vi "Dashboard.vi"() -> ()   [LabVIEW 2021]
uses:
  <vilib>/Instr/_visa.llb/VISA Configure Serial Port (Instr).vi
  <vilib>/addons/database/Connection.llb/DB Tools Open Connec (Path).vi
  <vilib>/addons/database/NI_Database_API.lvlib
panel:
  in  "Controle do alarme":dbl
  out "Alta Temperatura":bool
  out "TEMPERATURA [ºC]":dbl
  out "Temperatura":dbl(graph)
  out "ACELERADOR":dbl(graph)
  out "FREIO":dbl(graph)
  out "Temperatura":dbl(knob) caption="Meter" scale=0.0..120.0
  out "FREIO":u8(slide) scale=0.0..100.0
  out "ACELERADOR":u8(slide) scale=0.0..100.0
  out "ROTA敲O Z":dbl
  out "XY Graph 2":cluster{dbl, dbl}[](graph)
  out "GRAVIDADE (G)":dbl
  out "XY Graph":cluster{dbl, dbl}[](graph)
  out "read buffer":string
  out "result string":string
  in  "stop":bool
  in  "VISA resource name":refnum<visa-resource-name>
  # "Sátirus"
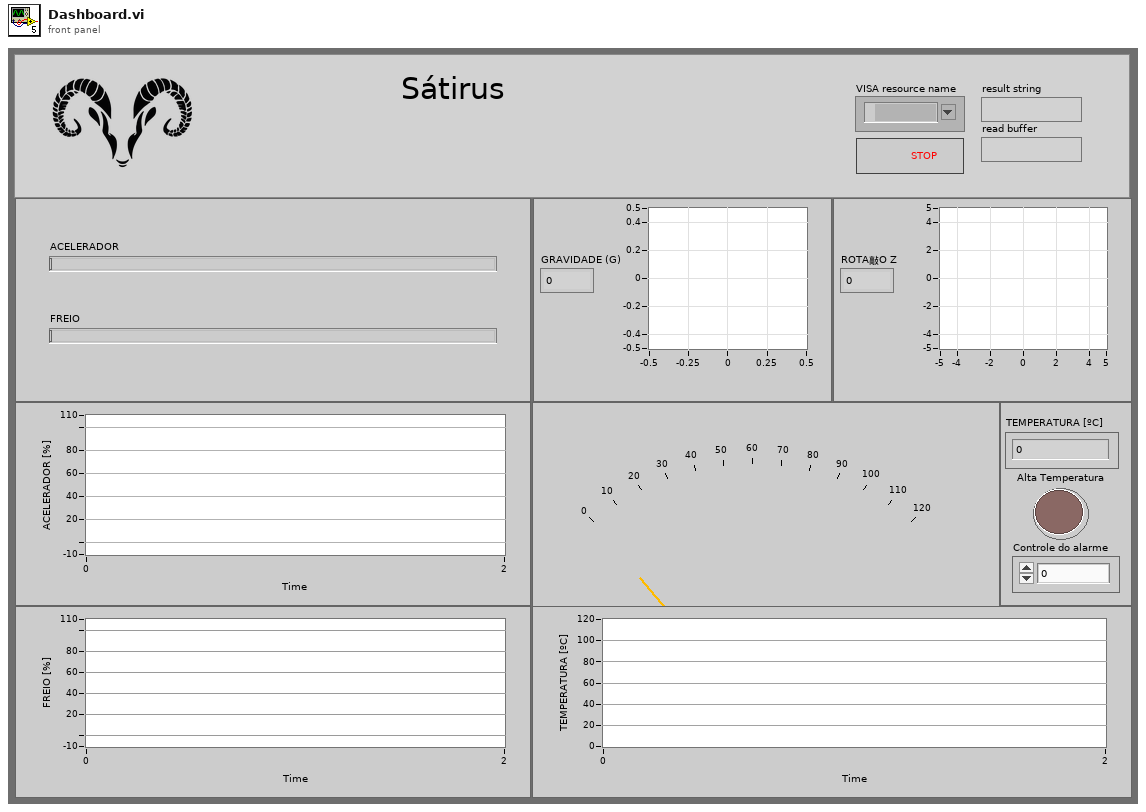
[diagram p1: front panel]
types:
  T1 = typedef "NI_Database_API.lvlib/Conn ObjectReference.ctl" = refnum<k1>
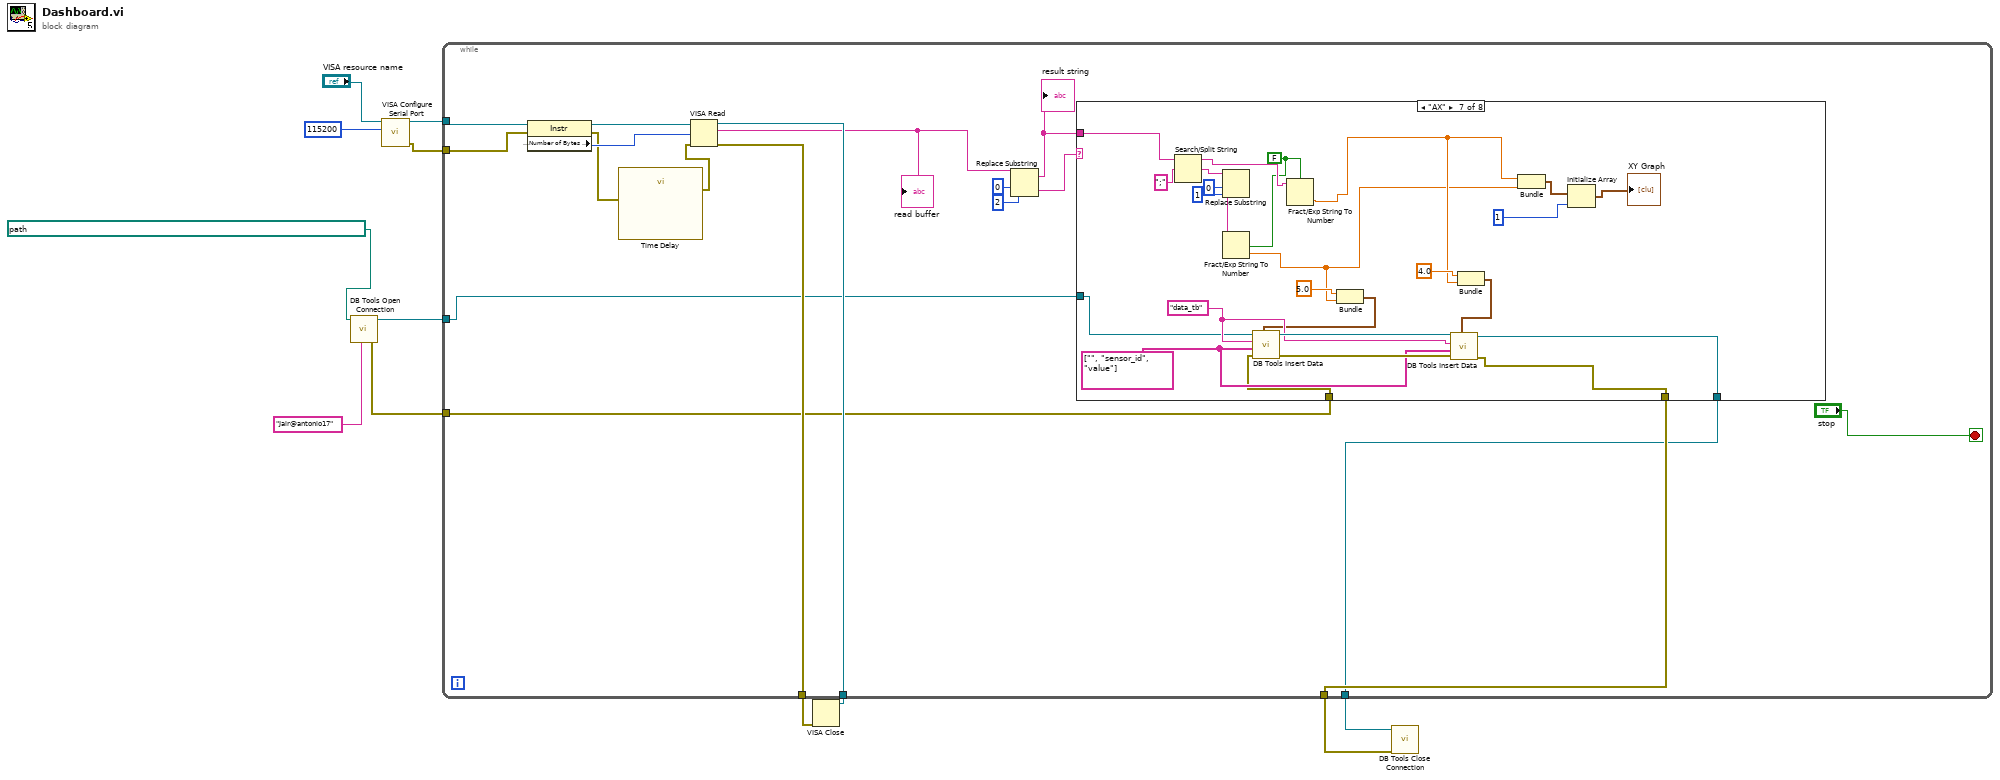
[diagram p0: block diagram]
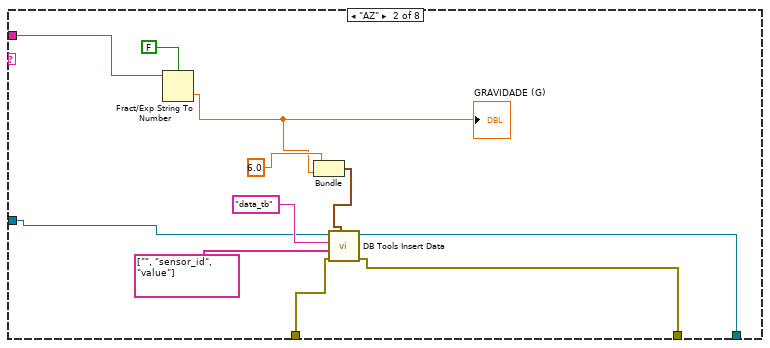
[diagram p3: hidden frame]
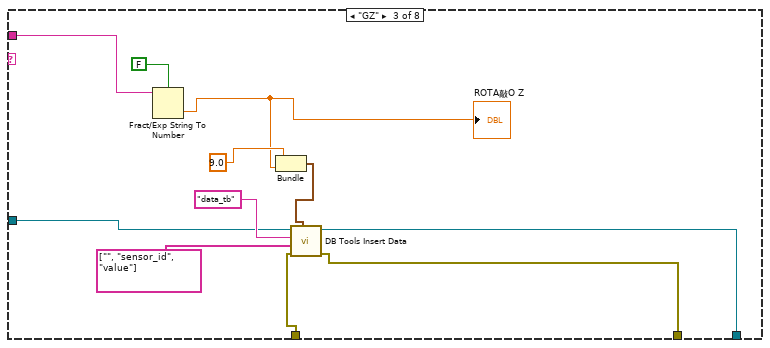
[diagram p4: hidden frame]
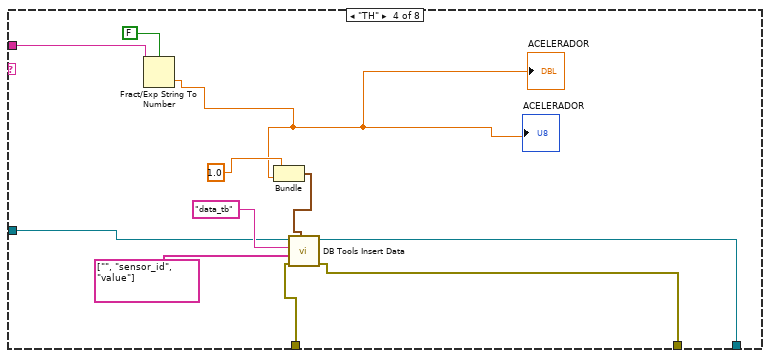
[diagram p5: hidden frame]
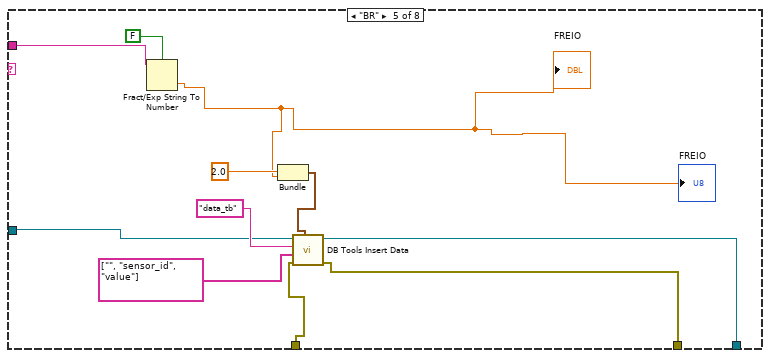
[diagram p6: hidden frame]
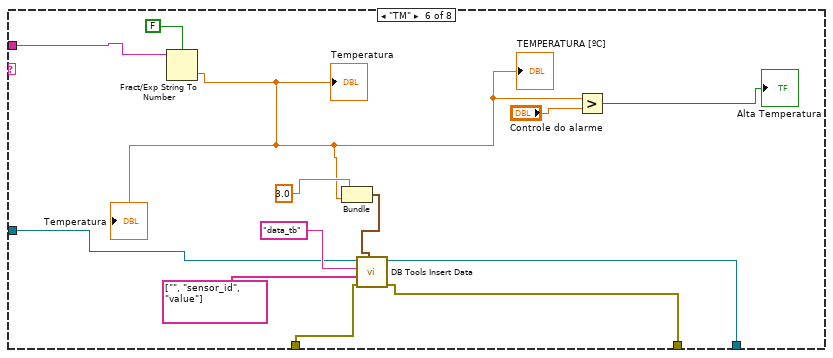
[diagram p7: hidden frame]
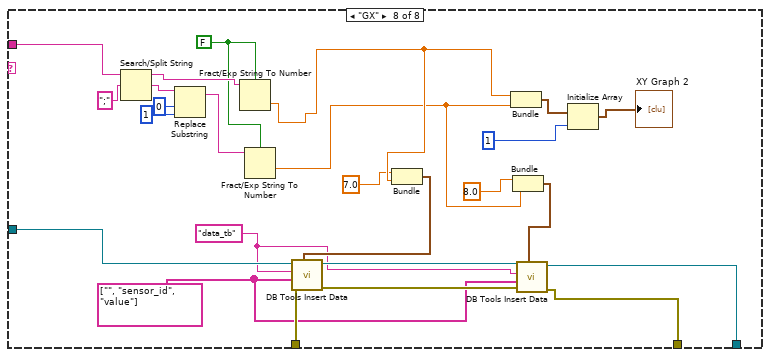
[diagram p8: hidden frame]
diagram:
  n1 = call-poly <vilib>:"DB Tools Open Connection.vi"("password"="Jair@antonio17", "connection information"=path "/\"C/Users/Usuário/Desktop/TCC/arquivos_tcc/DataBaseConectionFile.dsn\"" ("connection information 2")) -> ("error out"=w4:errorcluster, "connection reference"=w3:T1)  [unwired: 6 in]
  n2 = call-poly "VISA Configure Serial Port"("VISA resource name"="VISA resource name", "baud rate (9600)"=u32 115200) -> ("VISA resource name out"=w10:refnum<visa-resource-name>, "error out"=w9:errorcluster)  [unwired: 12 in]
  n3 = while {
    tunnel: w10 -> [w29]
    tunnel: w9 -> [w23]
    tunnel: [w30] -> w7
    tunnel: [w22] -> w8
    tunnel: w4 -> [w13]
    tunnel: w3 -> [w16]
    tunnel: [w15] -> w2
    tunnel: [w14] -> w1
    stop <- "stop" stop-if-true
    n4 = property class="Instr"(reference=w29, error in=w23) -> (reference out=w27:refnum<visa-resource-name>, error out=w18:errorcluster, "Serial Settings:Number of Bytes at Serial Port"=w28:u32)
    n5 = call "Time Delay"("error in (no error)"=w18) -> ("error out"=w17:errorcluster)  [unwired: 10 in]
    n6 = VISA Read(VISA resource name=w27, byte count=w28, error in (no error)=w17) -> (VISA resource name out=w30:refnum<visa-resource-name>, read buffer=w24:string, error out=w22:errorcluster)  [unwired: 1 out]
    "read buffer" <- w24
    n7 = Replace Substring(2:2 ("length (len. of substring)"), 3:0 ("offset (0)"), 5:w24) -> (0:w20:string, 1:w19:string)  [unwired: 1 in]
    "result string" <- w19
    n8 = case shown="\"AX\"" w20 {
      tunnel: w19 -> [_ w43 w54 w65 w76 w89 w108 w133]
      tunnel: w16 -> [w32 w37 w46 w60 w68 w80 w99 w128]
      tunnel: [w31 w35 w47 w56 w69 w78 w97 w123] -> w15
      tunnel: [w32 w34 w45 w55 w66 w77 w96 w122] -> w14
      tunnel: w13 -> [w31 w36 w48 w59 w70 w79 w98 w127]
      frame "False", Default {
      }
      frame "AZ" {
        n9 = Fract/Exp String To Number(use system decimal point (T)=FALSE, string=w43) -> (number=w33:dbl)  [unwired: 2 in, 1 out]
        "GRAVIDADE (G)" <- w33
        n10 = Bundle(6.0, w33) -> (w38:cluster{dbl, dbl})  [unwired: 1 in]
        n11 = call <vilib>:"DB Tools Insert Data.vi"("data"=w38, "error in (no error)"=w36, "columns"=string[] ["", "sensor_id", "value"], "table"="data_tb", "connection reference"=w37) -> ("error out"=w35:errorcluster, "connection reference out"=w34:T1)  [unwired: 5 in]
      }
      frame "GZ" {
        n12 = Fract/Exp String To Number(use system decimal point (T)=FALSE, string=w54) -> (number=w44:dbl)  [unwired: 2 in, 1 out]
        "ROTA敲O Z" <- w44
        n13 = Bundle(9.0, w44) -> (w49:cluster{dbl, dbl})  [unwired: 1 in]
        n14 = call <vilib>:"DB Tools Insert Data.vi"("data"=w49, "error in (no error)"=w48, "columns"=string[] ["", "sensor_id", "value"], "table"="data_tb", "connection reference"=w46) -> ("error out"=w47:errorcluster, "connection reference out"=w45:T1)  [unwired: 5 in]
      }
      frame "TH" {
        n15 = Fract/Exp String To Number(use system decimal point (T)=FALSE, string=w65) -> (number=w58:dbl)  [unwired: 2 in, 1 out]
        "ACELERADOR" <- w58
        "ACELERADOR" <- w58
        n16 = Bundle(1.0, w58) -> (w57:cluster{dbl, dbl})  [unwired: 1 in]
        n17 = call <vilib>:"DB Tools Insert Data.vi"("data"=w57, "error in (no error)"=w59, "columns"=string[] ["", "sensor_id", "value"], "table"="data_tb", "connection reference"=w60) -> ("error out"=w56:errorcluster, "connection reference out"=w55:T1)  [unwired: 5 in]
      }
      frame "BR" {
        n18 = Fract/Exp String To Number(use system decimal point (T)=FALSE, string=w76) -> (number=w67:dbl)  [unwired: 2 in, 1 out]
        "FREIO" <- w67
        "FREIO" <- w67
        n19 = Bundle(2.0, w67) -> (w74:cluster{dbl, dbl})  [unwired: 1 in]
        n20 = call <vilib>:"DB Tools Insert Data.vi"("data"=w74, "error in (no error)"=w70, "columns"=string[] ["", "sensor_id", "value"], "table"="data_tb", "connection reference"=w68) -> ("error out"=w69:errorcluster, "connection reference out"=w66:T1)  [unwired: 5 in]
      }
      frame "TM" {
        n21 = Fract/Exp String To Number(use system decimal point (T)=FALSE, string=w89) -> (number=w81:dbl)  [unwired: 2 in, 1 out]
        "Temperatura" <- w81
        "Temperatura" <- w81
        "TEMPERATURA [ºC]" <- w81
        n22 = Bundle(3.0, w81) -> (w82:cluster{dbl, dbl})  [unwired: 1 in]
        n23 = call <vilib>:"DB Tools Insert Data.vi"("data"=w82, "error in (no error)"=w79, "columns"=string[] ["", "sensor_id", "value"], "table"="data_tb", "connection reference"=w80) -> ("error out"=w78:errorcluster, "connection reference out"=w77:T1)  [unwired: 5 in]
        n24 = Greater?(x=w81, y="Controle do alarme") -> (0:→"Alta Temperatura":bool)
      }
      frame "AX" {
        w100 = string[] ["", "sensor_id", "value"] ("columns")
        w101 = "data_tb" ("table")
        w105 = FALSE ("use system decimal point (T)")
        n25 = Search/Split String(string=w108, search string/char (-)=";") -> (substring before match=w107:string, match + rest of string=w113:string)  [unwired: 1 in, 1 out]
        n26 = Replace Substring(2:1 ("length (len. of substring)"), 3:0 ("offset (0)"), 5:w113) -> (1:w106:string)  [unwired: 1 in, 1 out]
        n27 = Fract/Exp String To Number(use system decimal point (T)=w105, string=w106) -> (number=w90:dbl)  [unwired: 2 in, 1 out]
        n28 = Fract/Exp String To Number(use system decimal point (T)=w105, string=w107) -> (number=w93:dbl)  [unwired: 2 in, 1 out]
        n29 = Bundle(5.0, w90) -> (w91:cluster{dbl, dbl})  [unwired: 1 in]
        n30 = call <vilib>:"DB Tools Insert Data.vi"("data"=w91, "error in (no error)"=w98, "columns"=w100, "table"=w101, "connection reference"=w99) -> ("error out"=w102:errorcluster, "connection reference out"=w103:T1)  [unwired: 5 in]
        n31 = Bundle(4.0, w93) -> (w95:cluster{dbl, dbl})  [unwired: 1 in]
        n32 = call <vilib>:"DB Tools Insert Data.vi"("data"=w95, "error in (no error)"=w102, "columns"=w100, "table"=w101, "connection reference"=w103) -> ("error out"=w97:errorcluster, "connection reference out"=w96:T1)  [unwired: 5 in]
        n33 = Bundle(w93, w90) -> (w104:cluster{dbl, dbl})  [unwired: 1 in]
        n34 = Initialize Array(w104, 1 ("dimension size")) -> (→"XY Graph":cluster{dbl, dbl}[])
      }
      frame "GX" {
        w120 = string[] ["", "sensor_id", "value"] ("columns")
        w121 = "data_tb" ("table")
        w130 = FALSE ("use system decimal point (T)")
        n35 = Search/Split String(string=w133, search string/char (-)=";") -> (substring before match=w132:string, match + rest of string=w138:string)  [unwired: 1 in, 1 out]
        n36 = Replace Substring(2:1 ("length (len. of substring)"), 3:0 ("offset (0)"), 5:w138) -> (1:w131:string)  [unwired: 1 in, 1 out]
        n37 = Fract/Exp String To Number(use system decimal point (T)=w130, string=w132) -> (number=w118:dbl)  [unwired: 2 in, 1 out]
        n38 = Fract/Exp String To Number(use system decimal point (T)=w130, string=w131) -> (number=w115:dbl)  [unwired: 2 in, 1 out]
        n39 = Bundle(7.0, w118) -> (w126:cluster{dbl, dbl})  [unwired: 1 in]
        n40 = call <vilib>:"DB Tools Insert Data.vi"("data"=w126, "error in (no error)"=w127, "columns"=w120, "table"=w121, "connection reference"=w128) -> ("error out"=w124:errorcluster, "connection reference out"=w125:T1)  [unwired: 5 in]
        n41 = Bundle(w118, w115) -> (w129:cluster{dbl, dbl})  [unwired: 1 in]
        n42 = Bundle(8.0, w115) -> (w119:cluster{dbl, dbl})  [unwired: 1 in]
        n43 = call <vilib>:"DB Tools Insert Data.vi"("data"=w119, "error in (no error)"=w124, "columns"=w120, "table"=w121, "connection reference"=w125) -> ("error out"=w123:errorcluster, "connection reference out"=w122:T1)  [unwired: 5 in]
        n44 = Initialize Array(w129, 1 ("dimension size")) -> (→"XY Graph 2":cluster{dbl, dbl}[])
      }
    }
  }
  n45 = VISA Close(VISA resource name=w7, error in (no error)=w8) -> ()  [unwired: 1 out]
  n46 = call <vilib>:"DB Tools Close Connection.vi"("error in (no error)"=w2, "connection reference"=w1) -> ()  [unwired: 5 in, 1 out]
